vi "TCP send.vi"(8 "error in (no error)":errorcluster, 10 "string":string, 11 "connection ID in":refnum<k5>) -> (0 "error out":errorcluster, 3 "connection ID out":refnum<k5>)   [LabVIEW 2019]
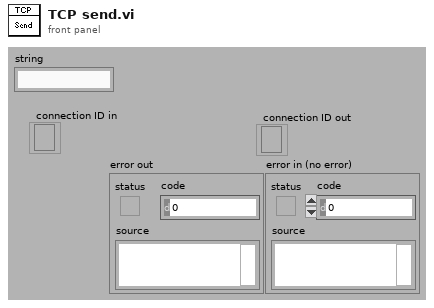
[diagram p1: front panel]
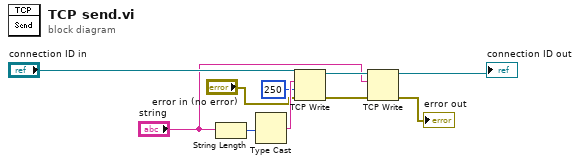
[diagram p0: block diagram]
diagram:
  n1 = String Length(string="string") -> (length=w10:i32)
  n2 = Type Cast(x=w10) -> (*(type *) &x=w6:string)  [unwired: 1 in]
  n3 = TCP Write(connection ID="connection ID in", data in=w6, error in (no error)="error in (no error)", 9:250 ("timeout ms (25000)")) -> (connection ID out=w7:refnum<k5>, error out=w5:errorcluster)  [unwired: 1 out]
  n4 = TCP Write(connection ID=w7, data in="string", error in (no error)=w5) -> (connection ID out=→"connection ID out":refnum<k5>, error out=→"error out":errorcluster)  [unwired: 1 in, 1 out]
